vi "Test Camera Image.vi"() -> ()   [LabVIEW 2014]
uses:
  Camera & Acquisition VIs/SubVIs/ctt's/Camera Setup Acquisition.ctl
  Camera & Acquisition VIs/SubVIs/ctt's/Image size and binning.ctl
  Camera & Acquisition VIs/SubVIs/ctt's/image-acquision 2.ctl
  Library Files - Andor and MadCity/Andorlib/atmcd32d.lvlib
panel:
  out "Image":T1(plugin-control)
  out "y size":u16
  out "x size":u16
  in  "stop":bool
  out "Image Array":u16[](array[numeric])
  in  "Image Size":T2={"H Bin"=1.0, "V Bin"=1.0, "Left"=1.0, "Right"=1024.0, "Top"=1.0, "Bottom"=1024.0} {"V Bin" min=0.0; "H Bin" min=0.0 step=1.0}
  in  "Acquisition Parameters":T3={"Readout Mode"=enum."Image", "Set Acquisition Mode"=enum."Single Scan", "Trigger Mode"=enum."Internal", "Exposure Time (sec)"=1.0, "Accumulation Cycle (s)"=1.0, "Kinetic Cycle Time (s)"=1.0, "Number of Kinetics"=1, "Number of Accumulations"=1, "Set VS Speed"=1.0, "Pixel Rate"=enum."Standard CCD 3 Mhz 14 bits", "V Shift Amplitude"=enum."+1", "Preamp Gain"=enum."1.0", "Single Track Settings"={"centre"=0, "height"=1}, "EM CCD Gain"=300, "High Capacity?"=FALSE} {"EM CCD Gain" scale=0.01..300.0; "Single Track Settings"."centre" min=0 max=1024; "Single Track Settings"."height" min=1 max=1024; "Exposure Time (sec)" scale=0.001..10.0 scale format="%#_1g"; "Set VS Speed" min=0.0 format="%#_2f"}
  # "****Configure Prior to Running Program****"
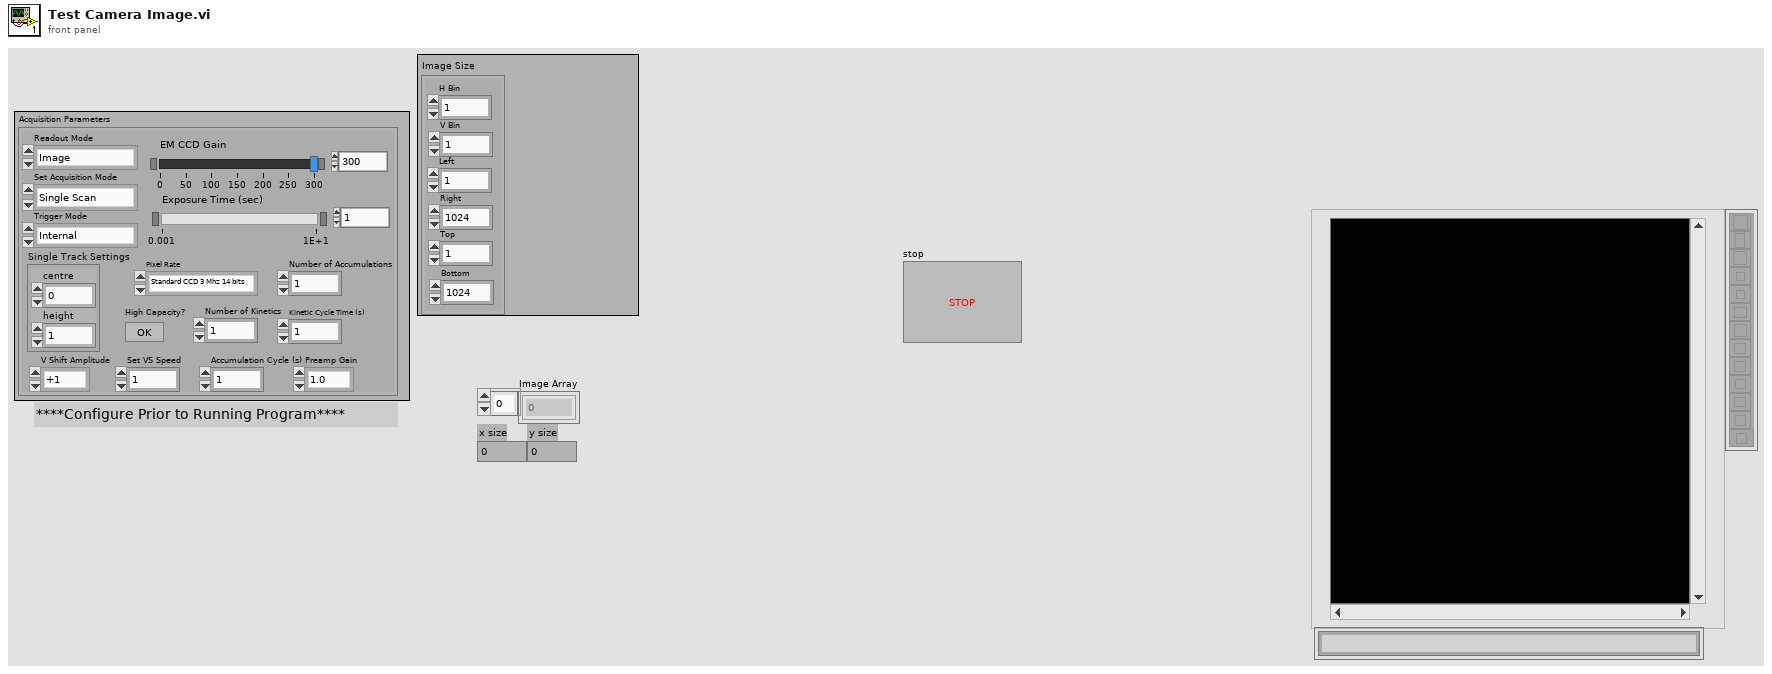
[diagram p1: front panel]
types:
  T1 = typedef "IMAQ Image.ctl" = refnum<image>
  T2 = typedef "Image size and binning.ctl" = cluster{"H Bin":dbl, "V Bin":dbl, "Left":dbl, "Right":dbl, "Top":dbl, "Bottom":dbl}
  T3 = typedef "Camera Setup Acquisition.ctl" = cluster{"Readout Mode":enum16{"Full Vertical Binning", "Multi-Track", "Random-Track", "Single-Track", "Image"}, "Set Acquisition Mode":enum16{"(do nothing)", "Single Scan", "Accumulate", "Kinetics", "Fast Kinetics", "Run till abort"}, "Trigger Mode":enum16{"Internal", "External"}, "Exposure Time (sec)":sgl, "Accumulation Cycle (s)":dbl, "Kinetic Cycle Time (s)":dbl, "Number of Kinetics":i32, "Number of Accumulations":i32, "Set VS Speed":dbl, "Pixel Rate":enum16{"EM CCD 10 Mhz 14 bits", "EM CCD 5 Mhz 14 bits", "EM CCD 3 Mhz 14 bits", "EM CCD 1 Mhz 16 bits", "Standard CCD 3 Mhz 14 bits", "Standard CCD 1 Mhz 16 bits"}, "V Shift Amplitude":enum16{"normal", "+1", "+2", "+3", "+4"}, "Preamp Gain":enum16{"1.0", "2.4", "5.0"}, "Single Track Settings":cluster{"centre":i32, "height":i32}, "EM CCD Gain":u16, "High Capacity?":bool}
  T4 = typedef "image-acquision 2.ctl" = u32
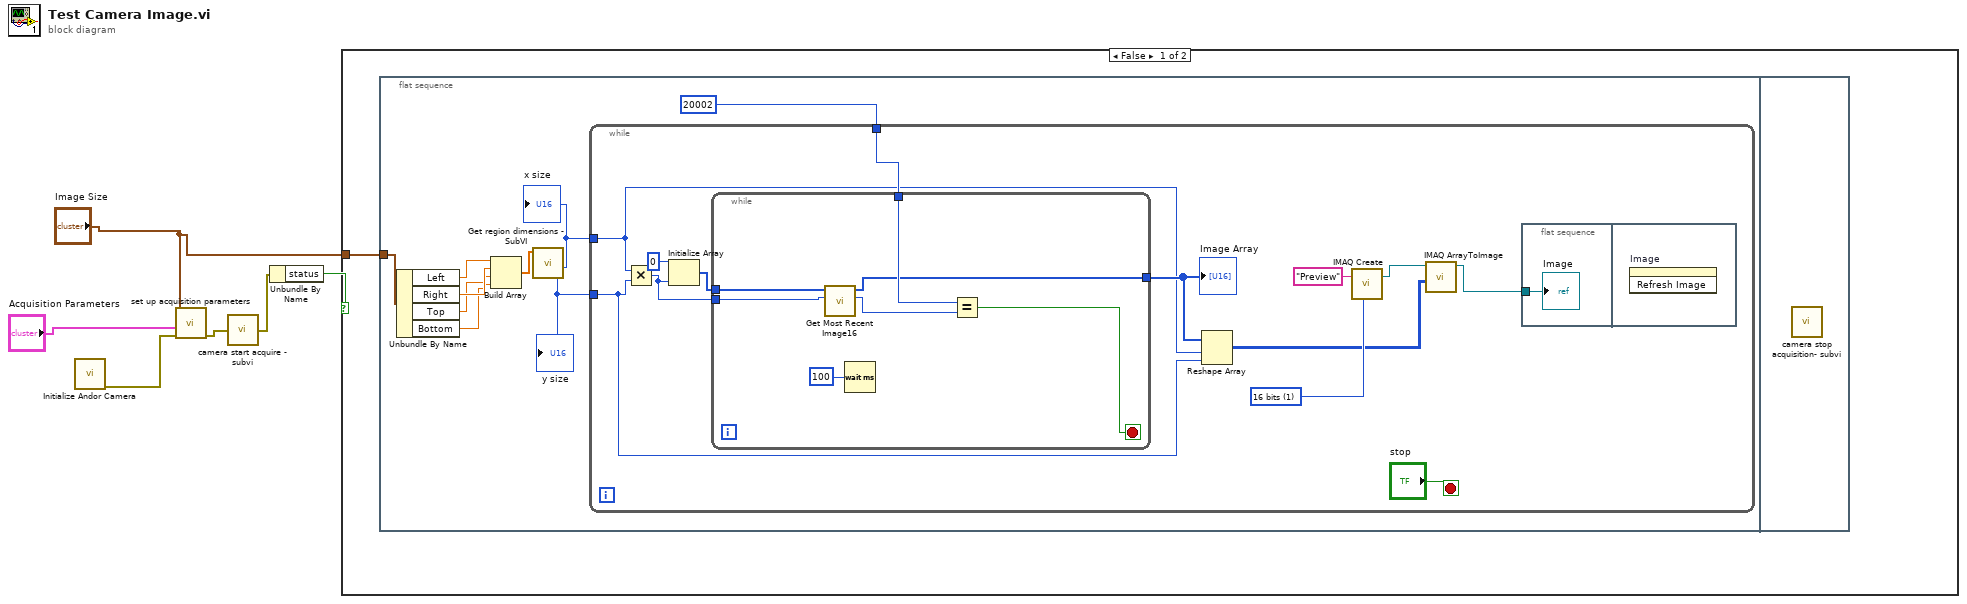
[diagram p0: block diagram]
diagram:
  n1 = call "Initialize Andor Camera.vi"() -> ("Error Out 2"=w6:errorcluster)  [unwired: 10 in, 1 out]
  n2 = call "set up acquisition parameters.vi"("error in (no error)"=w6, "Acquisition Parameters"="Acquisition Parameters", "Image Size"="Image Size") -> ("error out"=w5:errorcluster)  [unwired: 3 in, 3 out]
  n3 = call "camera start acquire - subvi.vi"("error in"=w5) -> ("error out"=w4:errorcluster)
  n4 = Unbundle By Name(w4) -> ("status"=w3:bool)
  n5 = case shown="False" w3 {
    tunnel: "Image Size" -> [w7 _]
    frame False {
      n6 = flat-sequence {
        tunnel: w7 -> [w15]
        frame #0 {
          n7 = Unbundle By Name(w15) -> ("Left"=w14:dbl, "Right"=w13:dbl, "Top"=w12:dbl, "Bottom"=w11:dbl)
          n8 = Build Array(w14, w13, w12, w11) -> (w10:dbl[])
          n9 = call "Get region dimensions - SubVI.vi"("x1y1x2y2"=w10) -> ("y size"=w8:u16, "x size"=w9:u16)  [unwired: 7 in, 2 out]
          "x size" <- w9
          "y size" <- w8
          n10 = while {
            tunnel: 20002 -> [w29]
            tunnel: w9 -> [w23]
            tunnel: w8 -> [w22]
            stop <- "stop" stop-if-true
            w19 = T4 1 items=["8 bits", "16 bits", "Float", "Complex", "RGB", "HSL"] ("Image Type")
            n11 = Multiply(x=w23, y=w22) -> (x*y=w24:u16)
            n12 = Initialize Array(u16 0 ("element"), w24) -> (w25:u16[])
            n13 = while {
              tunnel: w29 -> [w37]
              tunnel: [w33] -> w27
              tunnel: w25 -> [w32]
              tunnel: w24 -> [w31]
              stop <- w34 stop-if-true
              n14 = call "Get Most Recent Image16.vi"("size"=w31, "Array 2"=w32) -> ("function return"=w36:u32, "Array"=w33:u16[])  [unwired: 7 in, 1 out]
              n15 = Wait (ms)(milliseconds to wait=100) -> ()  [unwired: 1 out]
              n16 = Equal?(x=w37, y=w36) -> (x = y?=w34:bool)
            }
            "Image Array" <- w27
            n17 = Reshape Array(w27, w23, w22) -> (w18:u16[][])
            n18 = call "IMAQ Create"("Image Name"="Preview", "Image Type"=w19) -> ("New Image"=w20:T1)  [unwired: 3 in, 1 out]
            n19 = call "IMAQ ArrayToImage"("Image Pixels (I16)"=w18, "Image"=w20) -> ("Image Out"=w17:T1)  [unwired: 8 in, 1 out]
            n20 = flat-sequence {
              tunnel: w17 -> [w30]
              frame #0 {
                "Image" <- w30
              }
              frame #1 {
                n21 = invoke on="Image" class="ImageControl" method="Refresh Image"() -> ()  [unwired: 3 in, 3 out]
              }
            }
          }
        }
        frame #1 {
          n22 = call "camera stop acquisition- subvi.vi"() -> ()  [unwired: 1 in]
        }
      }
    }
    frame True {
    }
  }
